vi "Run Javascript.vi"(0 "Display State In":T1={"WebView2 Ref"=refnum, "event callback refnum"=refnum, "Events"={"Navigation Complete Event"=refnum, "Source Changed Event"=refnum, "Document Title Changed Event"=refnum, "Status Bar Text Changed"=refnum, "Web Message Received"=refnum, "Window Close Requested"=refnum}, "Paths"={"Webview2 Native"=path "C:/Users/kleins/Desktop/webview2/microsoft.web.webview2.1.0.1370.28/build/native", "Edge Application"=path "", "User Data"=path ""}}, 5 "javaScript":string, 9 "Container State":T3, 11 "error in (no error)":errorcluster) -> (4 "Display State Out":T1={"WebView2 Ref"=refnum, "event callback refnum"=refnum, "Events"={"Navigation Complete Event"=refnum, "Source Changed Event"=refnum, "Document Title Changed Event"=refnum, "Status Bar Text Changed"=refnum, "Web Message Received"=refnum, "Window Close Requested"=refnum}, "Paths"={"Webview2 Native"=path "C:/Users/kleins/Desktop/webview2/microsoft.web.webview2.1.0.1370.28/build/native", "Edge Application"=path "", "User Data"=path ""}}, 15 "error out":errorcluster)   [LabVIEW 2020, in "WebView2 Control.xctl"]
uses:
  WebView2 Control.xctl
  <vilib>/_xctls/Container State.ctl
  State.ctl
  C:/Users/kleins/Desktop/webview2/microsoft.web.webview2.1.0.1370.28/lib/net45/Microsoft.Web.WebView2.WinForms.dll
  microsoft.web.webview2.1.0.1370.28/lib/net45/Microsoft.Web.WebView2.WinForms.dll
  Paths.ctl
  C:/Users/kleins/Desktop/webview2/microsoft.web.webview2.1.0.1370.28/lib/net45/Microsoft.Web.WebView2.Core.dll
  microsoft.web.webview2.1.0.1370.28/lib/net45/Microsoft.Web.WebView2.Core.dll
  <vilib>/_xctls/XControlSupport.lvlib
panel:
  # "Add Controls & Indicators that form the parameters of the method here. Hook them to the connector pane. Do not delete the controls & indicators that are already hooked to the connector pane.\n \nTo setup the parameters  for this method, right click on this item in the Project Tree & select \"Configure Method...\"."
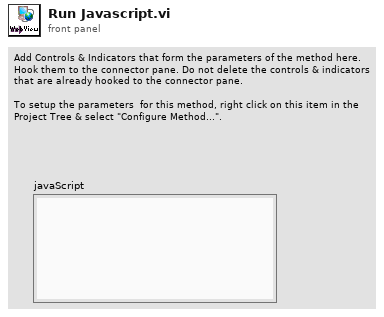
[diagram p1: front panel]
types:
  T1 = typedef "WebView2 Control.xctl/State.ctl" = cluster{"WebView2 Ref":refnum<data-value>, "event callback refnum":refnum<k27>, "Events":cluster{"Navigation Complete Event":refnum<user-event>, "Source Changed Event":refnum<user-event>, "Document Title Changed Event":refnum<user-event>, "Status Bar Text Changed":refnum<user-event>, "Web Message Received":refnum<user-event>, "Window Close Requested":refnum<user-event>}, "Paths":T2}
  T2 = typedef "WebView2 Control.xctl/Paths.ctl" = cluster{"Webview2 Native":path, "Edge Application":path, "User Data":path}
  T3 = typedef "XControlSupport.lvlib/Container State.ctl" = cluster{"Indicator?":bool, "Run Mode?":bool, " Refnum":refnum<vi>}
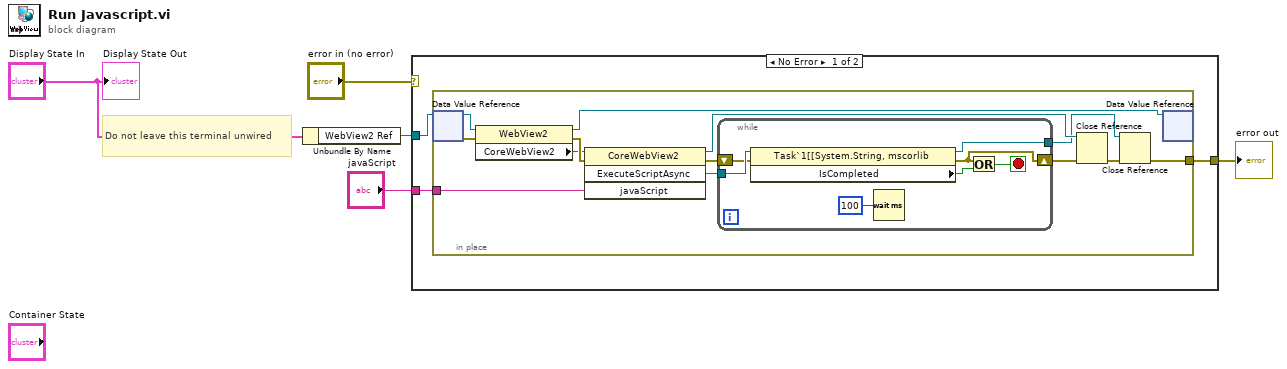
[diagram p0: block diagram]
diagram:
  # "Do not leave this terminal unwired"
  n1 = Unbundle By Name("Display State In") -> ("WebView2 Ref"=w5:refnum<data-value>)
  n2 = case shown="No Error" "error in (no error)" {
    selector: "error in (no error)" -> [_ w29]
    tunnel: [w8 w29] -> w1
    tunnel: w5 -> [w7 _]
    tunnel: "javaScript" -> [w6 _]
    frame No Error {
      n3 = in-place {
        in-place-border: [w10] -> w8
        in-place-border: w6 -> [w14]
        n4 = in-place-dvr #1(w7) -> (w20:refnum<k24>, w19:errorcluster)
        n5 = property class="WebView2"(reference=w20, error in=w19) -> (reference out=w18:refnum<k24>, error out=w21:errorcluster, "CoreWebView2"=w15:refnum<k24>)
        n6 = invoke class="CoreWebView2" method="ExecuteScriptAsync"(reference=w15, error in=w21, "javaScript"=w14) -> (reference out=w16:refnum<k24>, error out=w12:errorcluster, "ExecuteScriptAsync"=w13:refnum<k24>)  [unwired: 1 in, 1 out]
        n7 = while {
          tunnel: w13 -> [w28]
          shift-right: [w26] -> w11
          shift-left: w12 -> [w27]
          tunnel: [w22] -> w9
          stop <- w25 stop-if-true
          n8 = property class="Task`1[[System.String, mscorlib"(reference=w28, error in=w27) -> (reference out=w22:refnum<k24>, error out=w26:errorcluster, "IsCompleted"=w24:bool)
          n9 = Wait (ms)(milliseconds to wait=u32 100) -> ()  [unwired: 1 out]
          n10 = Or(x=w26, y=w24) -> (x .or. y?=w25:bool)
        }
        n11 = Close Reference(reference=w16, error in (no error)=w11) -> (error out=w17:errorcluster)
        n12 = Close Reference(reference=w9, error in (no error)=w17) -> (error out=w10:errorcluster)
        n13 = in-place-dvr #1(w18) -> ()  [unwired: 2 out]
      }
    }
    frame Error {
    }
  }
  "error out" <- w1
  "Display State Out" <- "Display State In"
